vi "Periodic Tasks.vi"(8 "error in":errorcluster) -> ()   [LabVIEW 2016]
doc: "This VI runs in parallel to other tasks. It can contain as many user-defined periodic loops as you need. These can carry out PID or other sorts of timed response."
uses:
  <vilib>/Rock Robotics/WPI/Utilities/WPI_GetSetVariantRefNum.vi
  Robot Global Data.vi
  <vilib>/Rock Robotics/Network Tables/NT Read Boolean.vi
  <vilib>/Rock Robotics/Network Tables/NT Read Number.vi
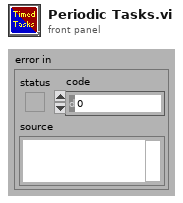
[diagram p1: front panel]
types:
  T1 = typedef "WPI_JoystickDevRef.ctl" = cluster{"Device":T2}
  T2 = typedef "WPI_JoystickDeviceEnum.ctl" = enum16{"USB 0", "USB 1", "USB 2", "USB 3", "USB 4", "USB 5"}
  T3 = typedef "WPI_RobotDriveDevRef.ctl" = cluster{"DevStatus":errorcluster, "Motors[]":T4[], "Square Inputs":bool, "Max Output":dbl}
  T4 = typedef "WPI_MotorControlDeviceRef.ctl" = cluster{"DeviceStatus":errorcluster, "Type":T5, "PWM":cluster{"PWM Channel":T6, "DeadBand":T7}, "CAN":cluster{"Device Number":u8, "SetOutput VI Ref":variant, "GetOutput VI Ref":variant, "Enable VI Ref":variant, "Disable VI Ref":variant, "Data":variant}, "Invert":bool}
  T5 = typedef "WPI_MotorControlType.ctl" = enum16{"PWM", "CAN"}
  T6 = typedef "FPGA_DIOPWMChannel.ctl" = enum8{"PWM 0", "PWM 1", "PWM 2", "PWM 3", "PWM 4", "PWM 5", "PWM 6", "PWM 7", "PWM 8", "PWM 9", "PWM MXP 0", "PWM MXP 1", "PWM MXP 2", "PWM MXP 3", "PWM MXP 4", "PWM MXP 5", "PWM MXP 6", "PWM MXP 7", "PWM MXP 8", "PWM MXP 9", "Invalid"}
  T7 = typedef "WPI_PWMDeadband.ctl" = cluster{"Name":string, "maxPositivePwm":i32, "minPositivePwm":i32, "centerPwm":i32, "maxNegativePwm":i32, "minNegativePwm":i32, "angularRange":u16}
  T8 = cluster{"JoystickDevRef":T1, "RobotDriveDevRef":T3}
  T9 = typedef "WPI_ServoDeviceRef.ctl" = cluster{"DeviceStatus":errorcluster, "PWM Channel":T6, "DeadBand":T7}
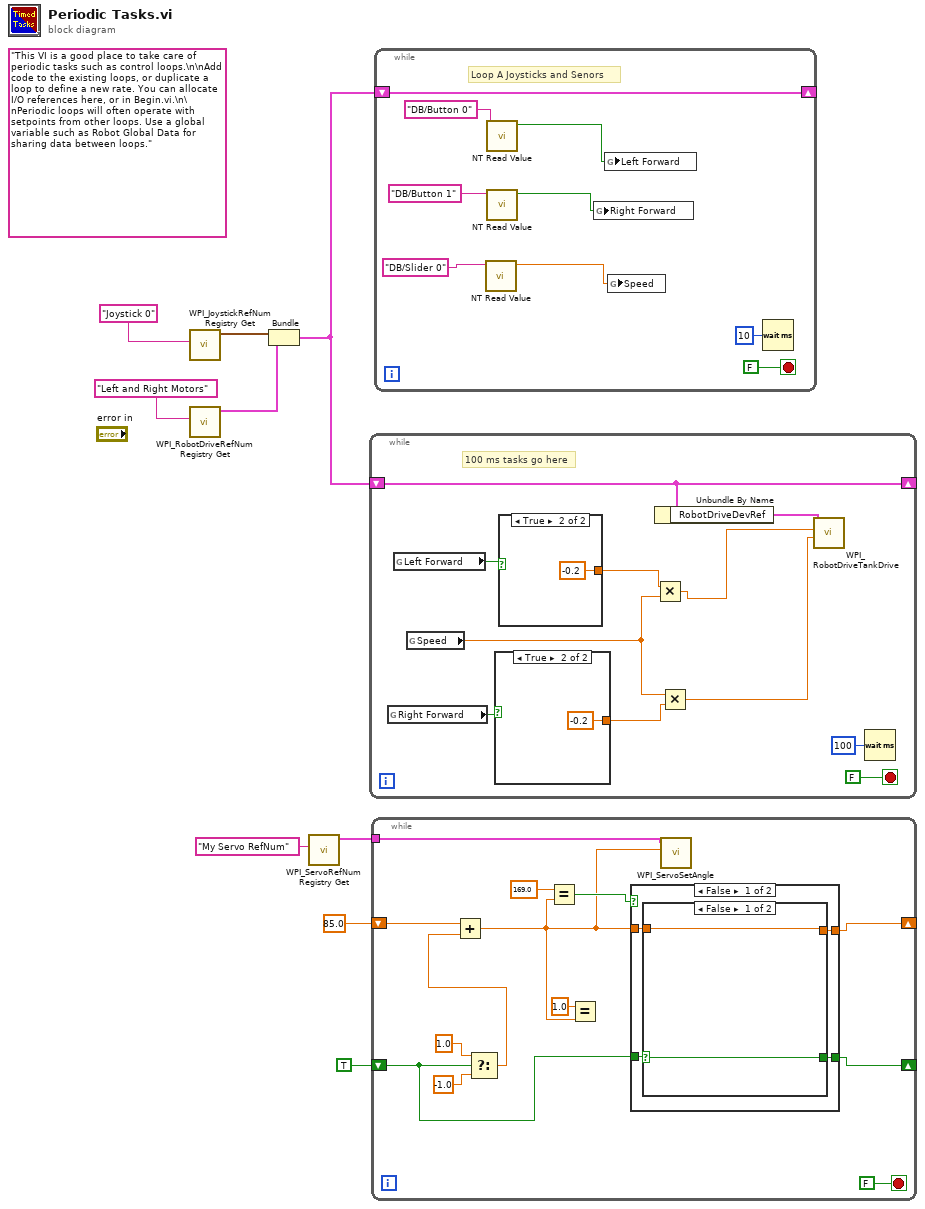
[diagram p0: block diagram]
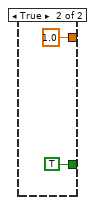
[diagram p2: hidden frame]
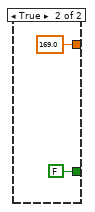
[diagram p3: hidden frame]
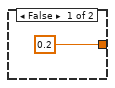
[diagram p4: hidden frame]
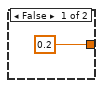
[diagram p5: hidden frame]
diagram:
  (unwired) "This VI is a good place to take care of periodic tasks such as control loops.\n\nAdd code to the existing loops, or duplicate a loop to define a new rate. You can allocate I/O references here, or in Begin.vi.\n\nPeriodic loops will often operate with setpoints from other loops. Use a global variable such as Robot Global Data for sharing data between loops."
  n1 = call <vilib>:"WPI_JoystickRefNum Registry Get.vi"("refnum name"="Joystick 0") -> ("JoystickDevRef"=w7:T1)  [unwired: 1 in, 9 out]
  n2 = call <vilib>:"WPI_RobotDriveRefNum Registry Get.vi"("refnum name"="Left and Right Motors") -> ("RobotDriveDevRef"=w6:T3)  [unwired: 1 in, 9 out]
  n3 = Bundle("JoystickDevRef"=w7, "RobotDriveDevRef"=w6) -> (w5:T8)  [unwired: 1 out]
  n4 = call <vilib>:"WPI_ServoRefNum Registry Get.vi"("refnum name"="My Servo RefNum") -> ("ServoDeviceRef"=w2:T9)  [unwired: 9 in, 1 out]
  n5 = while {
    shift-right: [w13] -> _
    shift-left: w5 -> [w13]
    stop <- FALSE stop-if-true
    # "100 ms tasks go here"
    n6 = global read "Robot Global Data.vi" "Right Forward"() -> (w17:bool)
    n7 = global read "Robot Global Data.vi" "Left Forward"() -> (w18:bool)
    n8 = global read "Robot Global Data.vi" "Speed"() -> (w14:dbl)
    n9 = case shown="True" w17 {
      tunnel: [0.2 ("Speed") -0.2 ("Speed")] -> w15
      frame False {
      }
      frame True {
      }
    }
    n10 = case shown="True" w18 {
      tunnel: [0.2 ("Speed") -0.2 ("Speed")] -> w16
      frame False {
      }
      frame True {
      }
    }
    n11 = Unbundle By Name(w13) -> ("RobotDriveDevRef"=w12:T3)
    n12 = Multiply(x=w16, y=w14) -> (x*y=w11:dbl)
    n13 = Multiply(x=w14, y=w15) -> (x*y=w10:dbl)
    n14 = call <vilib>:"WPI_RobotDriveTankDrive.vi"("Right axis value"=w10, "Left axis value"=w11, "RobotDriveDevRef"=w12) -> ()  [unwired: 6 in, 3 out]
    n15 = Wait (ms)(milliseconds to wait=u32 100) -> ()  [unwired: 1 out]
  }
  n16 = while {
    shift-right: [w28] -> _
    shift-left: 85.0 ("x") -> [w37]
    shift-right: [w27] -> _
    shift-left: TRUE ("s") -> [w32]
    tunnel: w2 -> [w26]
    stop <- FALSE stop-if-true
    n17 = Select(t=1.0, s=w32, f=-1.0) -> (s? t:f=w33:dbl)
    n18 = Add(x=w37, y=w33) -> (x+y=w25:dbl)
    n19 = Equal?(x=169.0, y=w25) -> (x = y?=w29:bool)
    n20 = Equal?(x=1.0, y=w25) -> ()  [unwired: 1 out]
    n21 = case shown="False" w29 {
      tunnel: w32 -> [w41 _]
      tunnel: w25 -> [w40 _]
      tunnel: [w39 169.0] -> w28
      tunnel: [w38 FALSE] -> w27
      frame False {
        n22 = case shown="False" w41 {
          selector: w41 -> [w42 _]
          tunnel: [w43 1.0] -> w39
          tunnel: w40 -> [w43 _]
          tunnel: [w42 TRUE] -> w38
          frame False {
          }
          frame True {
          }
        }
      }
      frame True {
      }
    }
    n23 = call <vilib>:"WPI_ServoSetAngle.vi"("Angle"=w25, "ServoDeviceRef"=w26) -> ()  [unwired: 8 in, 2 out]
  }
  n24 = while {
    shift-right: [w54] -> _
    shift-left: w5 -> [w54]
    stop <- FALSE stop-if-true
    # "Loop A Joysticks and Senors"
    n25 = call-poly <vilib>:"NT Read Value.vi"("Name"="DB/Slider 0") -> ("Numeric"=w48:dbl)  [unwired: 9 in, 1 out]
    n26 = call-poly <vilib>:"NT Read Value.vi"("Name"="DB/Button 0") -> ("Boolean"=w50:bool)  [unwired: 9 in, 1 out]
    n27 = call-poly <vilib>:"NT Read Value.vi"("Name"="DB/Button 1") -> ("Boolean"=w49:bool)  [unwired: 9 in, 1 out]
    n28 = global write "Robot Global Data.vi" "Right Forward"(w49) -> ()
    n29 = global write "Robot Global Data.vi" "Left Forward"(w50) -> ()
    n30 = global write "Robot Global Data.vi" "Speed"(w48) -> ()
    n31 = Wait (ms)(milliseconds to wait=u32 10) -> ()  [unwired: 1 out]
  }
